vi "Spawn Process.vi"(8 "error in (no error)":errorcluster, 11 "Test Manager in":refnum<class "Basic Test Manager.lvclass">) -> (0 "error out":errorcluster, 3 "Test Manager out":refnum<class "Basic Test Manager.lvclass">)   [LabVIEW 2009, in "Caraya.lvlib" / "Basic Test Manager.lvclass"]
uses:
  Basic Test Manager.lvclass
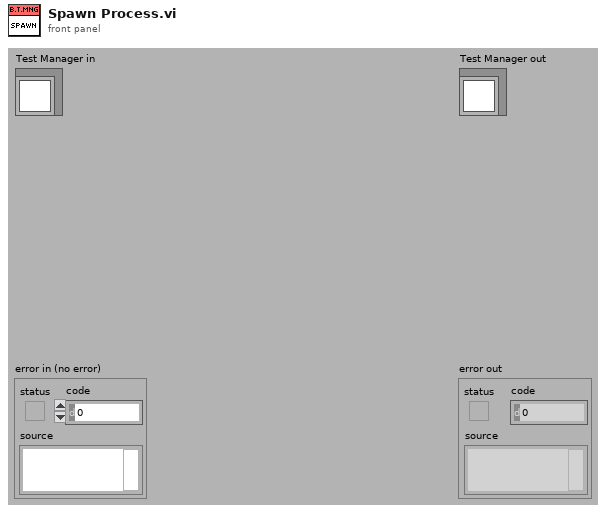
[diagram p1: front panel]
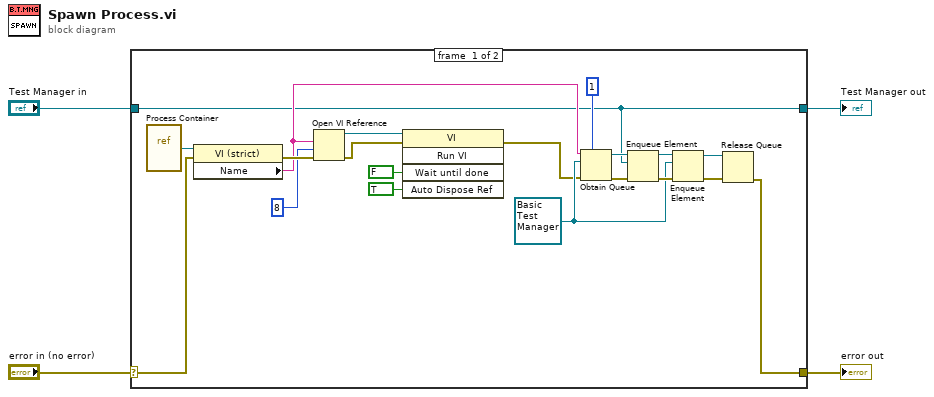
[diagram p0: block diagram]
diagram:
  n1 = case shown="No Error" "error in (no error)" {
    selector: "error in (no error)" -> [w18 w26]
    tunnel: [w8 w26] -> w3
    tunnel: [w13 w25] -> w1
    tunnel: "Test Manager in" -> [w13 w25]
    frame #0 {
      w7 = refnum<class "Basic Test Manager.lvclass"> refnum ("element")
      n2 = vi-ref "Process Container.vi"() -> (w23:refnum<vi>)
      n3 = property class="VI (strict)"(reference=w23, error in=w18) -> (error out=w24:errorcluster, "Name"=w17:string)  [unwired: 1 out]
      n4 = Open VI Reference(vi path=w17, options=8, error in (no error)=w24) -> (vi reference=w21:refnum<vi>, error out=w22:errorcluster)  [unwired: 3 in]
      n5 = invoke class="VI" method="Run VI"(reference=w21, error in=w22, "Wait until done"=FALSE ("Wait Until Done"), "Auto Dispose Ref"=TRUE ("Auto Dispose Reference")) -> (error out=w5:errorcluster)  [unwired: 1 in, 4 out]
      n6 = Obtain Queue(max queue size (-1, unlimited)=1, name (unnamed)=w17, element data type=w7, error in (no error)=w5) -> (queue out=w15:refnum<queue>, error out=w14:errorcluster)  [unwired: 1 in, 1 out]
      n7 = Enqueue Element(queue=w15, element=w13, error in (no error)=w14) -> (queue out=w12:refnum<queue>, error out=w11:errorcluster)  [unwired: 1 in, 1 out]
      n8 = Enqueue Element(queue=w12, element=w7, error in (no error)=w11) -> (queue out=w10:refnum<queue>, error out=w9:errorcluster)  [unwired: 1 in, 1 out]
      n9 = Release Queue(queue=w10, error in (no error)=w9) -> (error out=w8:errorcluster)  [unwired: 1 in, 2 out]
    }
    frame #1 {
    }
  }
  "error out" <- w3
  "Test Manager out" <- w1
